vi "Emballage_BDD_lectureSQL_Liste PièceDansCmd.vi"(6 "order by":string="DATE_EMBALLAGE", 8 "Error in":errorcluster caption="Error in (no error)", 9 "Colonnes":string[](array[string])=["SN_PRODUIT\n", "DATE_EMBALLAGE\n", "ID_UTILISATEUR_GPAO\n", "NO_CDEVAL\n", "NO_DU_CARTON\n", "NO_RETOUR_CLIENT\n"], 10 "NO_CDEVAL":string="6340/07-02.01.01", 11 "Table (PRODUIT_EMBALLAGE)":string="PRODUIT_EMBALLAGE") -> (0 "Error out":errorcluster, 1 "Erreur de  comunication":bool, 2 "Liste n° pièces de la cmde":string[](array[string]), 3 "Donnees":string[][](array[string]), 4 "Carton":string[](array[string]))   [LabVIEW 2020]
uses:
  Modules/FS/60_FS_Controles/60_FS_SetGet.ctl
  <vilib>/addons/database/Connection.llb/DB Tools Open Connec (Path).vi
  <vilib>/addons/database/Connection.llb/Conn Execute.vi
  <vilib>/addons/database/Recordset.llb/Rec Fetch Recordset Data (R).vi
  <vilib>/addons/database/Recordset.llb/Rec Destroy - Connection.vi
  <vilib>/addons/database/NI_Database_API.lvlib
panel:
  out "temps Exe [s]":dbl
  in  "En cas de retour":string
  # "0"
  # "5"
  # "1"
  # "2"
  # "3"
  # "4"
  # "#LTI 20180802\nC'est quoi??\nvoir ancien et pas utiliser"
  # "0: SN_PRODUIT\n1: DATE_EMBALLAGE\n2: ID_UTILISATEUR_GPAO\n3: NO_CDEVAL\n4: NO_DU_CARTON\n5: NO_RETOUR_CLIENT"
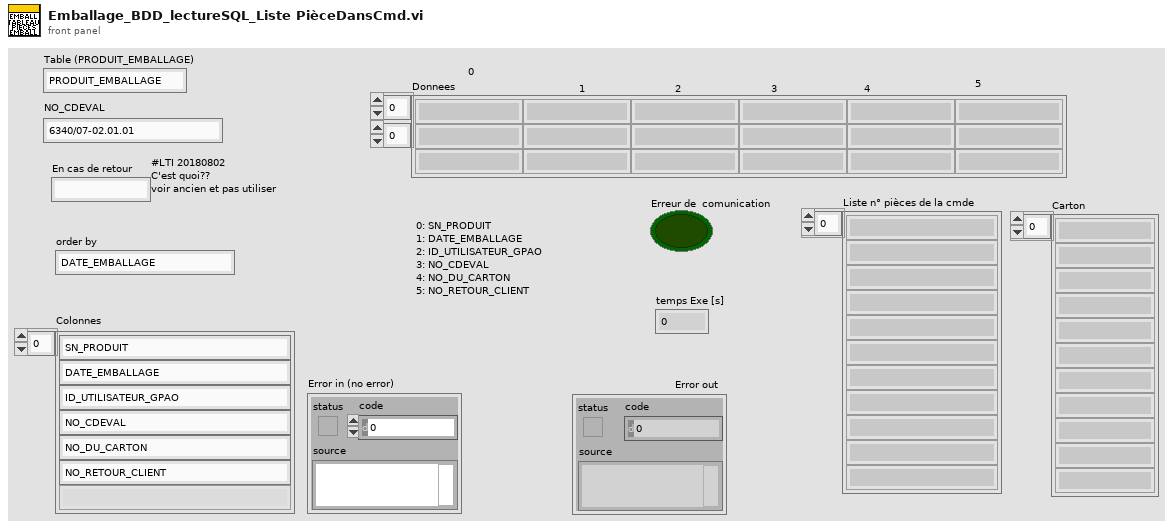
[diagram p1: front panel]
types:
  T1 = typedef "60_FS_SetGet.ctl" = enum16{"set", "get"}
  T2 = typedef "60_FS_CLT_Chemins.ctl" = cluster{"Racine_local":path, "Racine_reseau":path, "Racine_Support_Application":path, "Fichier_Journalisation":path, "Connexion_BDD_VSX":path, "Connexion_BDD_PLZ":path}
  T3 = typedef "NI_Database_API.lvlib/Conn ObjectReference.ctl" = refnum<k1>
  T4 = typedef "NI_Database_API.lvlib/Rec ObjectReference.ctl" = refnum<k1>
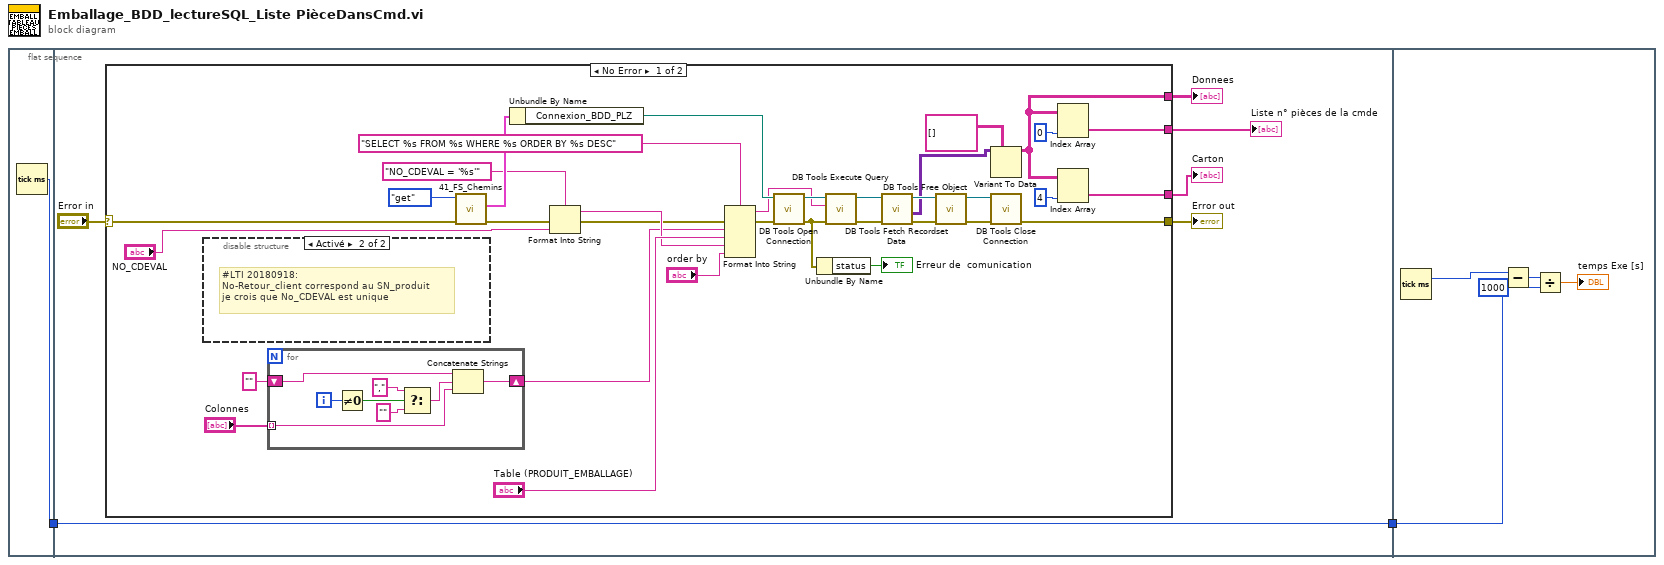
[diagram p0: block diagram]
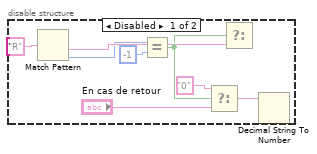
[diagram p2: hidden frame]
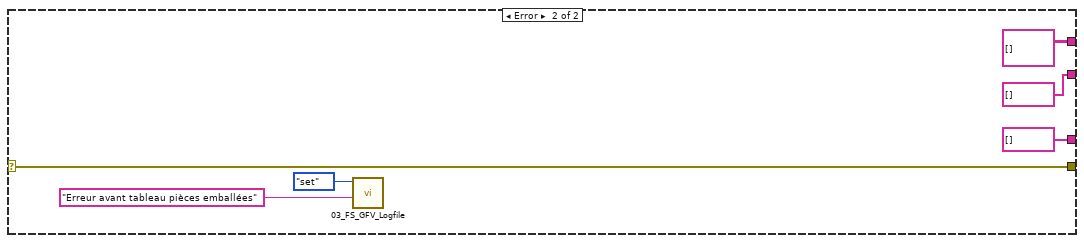
[diagram p3: hidden frame]
diagram:
  n1 = flat-sequence {
    tunnel: [w3] -> w2
    tunnel: w2 -> [w4]
    tunnel: [w4] -> w1
    tunnel: w1 -> [w66]
    frame #0 {
      n2 = Tick Count (ms)() -> (millisecond timer value=w3:u32)
    }
    frame #1 {
      n3 = case shown="No Error" "Error in" {
        selector: "Error in" -> [w29 w65]
        tunnel: [w28 w65] -> w8
        tunnel: [w12 string[][] [] ("Liste des champs à lire 2")] -> w7
        tunnel: [w14 string[] [] ("Liste des champs à lire 2")] -> w5
        tunnel: [w11 string[] [] ("Liste des champs à lire 2")] -> w6
        frame No Error {
          n4 = disable-structure shown="Activé" {
            frame Disabled {
              n5 = Match Pattern(regular expression="R" ("expression régulière")) -> (after substring=w51:string, offset past match=w49:i32)  [unwired: 2 in, 2 out]
              n6 = Equal?(x=w49, y=-1) -> (x = y?=w46:bool)
              n7 = Select(t="0", s=w46, f="En cas de retour") -> (s? t:f=w44:string)
              n8 = Select(s=w46, f=w51) -> ()  [unwired: 1 in, 1 out]
              n9 = Decimal String To Number(string=w44) -> ()  [unwired: 2 in, 2 out]
            }
            frame Enabled {
              # "#LTI 20180918:\nNo-Retour_client correspond au SN_produit\nje crois que No_CDEVAL est unique"
            }
          }
          n10 = for {
            tunnel: "Colonnes" -> [w58] mode=indexing
            shift-right: [w59] -> w19
            shift-left: "" -> [w57]
            i -> [w56]
            n11 = Not Equal To 0?(x=w56) -> (x != 0?=w55:bool)
            n12 = Select(t="," ("cas vrai"), s=w55, f="") -> (s? t:f=w54:string)
            n13 = Concatenate Strings(w57, w54, w58) -> (w59:string)
          }
          n14 = call "41_FS_Chemins.vi"("error in (no error)"=w29, "SetGet"=60_FS_SetGet."get") -> ("error out"=w31:errorcluster, "CLT_Chemins_out"=w39:T2)  [unwired: 8 in]
          n15 = Unbundle By Name(w39) -> ("Connexion_BDD_PLZ"=w37:path)
          n16 = Format Into String(format string="NO_CDEVAL = '%s'" ("chaîne de format"), error in=w31, "NO_CDEVAL") -> (resulting string=w33:string, error out=w30:errorcluster)  [unwired: 1 in]
          n17 = Format Into String(format string="SELECT %s FROM %s WHERE %s ORDER BY %s DESC" ("chaîne de format"), error in=w30, w19, "Table (PRODUIT_EMBALLAGE)", w33, "order by") -> (resulting string=w34:string, error out=w40:errorcluster)  [unwired: 1 in]
          n18 = call-poly <vilib>:"DB Tools Open Connection.vi"("error in (no error)"=w40, "connection information"=w37) -> ("error out"=w17:errorcluster, "connection reference"=w41:T3)  [unwired: 6 in]
          n19 = Unbundle By Name(w17) -> ("status"=→"Erreur de  comunication":bool)
          n20 = call-poly <vilib>:"DB Tools Execute Query.vi"("error in (no error)"=w17, "SQL query"=w34, "connection reference"=w41) -> ("error out"=w27:errorcluster, "recordset reference"=w25:T4)  [unwired: 5 in]
          n21 = call-poly <vilib>:"DB Tools Fetch Recordset Data.vi"("error in (no error)"=w27, "recordset reference"=w25) -> ("error out"=w26:errorcluster, "recordset data"=w23:variant[][], "recordset reference out"=w24:T4)  [unwired: 3 in]
          n22 = call-poly <vilib>:"DB Tools Free Object.vi"("error in (no error)"=w26, "recordset reference"=w24) -> ("error out"=w43:errorcluster, "connection reference"=w42:T3)  [unwired: 8 in]
          n23 = Variant To Data(type=string[][] [] ("Liste des champs à lire 2"), Variant=w23) -> (data=w12:string[][])  [unwired: 1 in, 1 out]
          n24 = call <vilib>:"DB Tools Close Connection.vi"("error in (no error)"=w43, "connection reference"=w42) -> ("error out"=w28:errorcluster)  [unwired: 5 in]
          n25 = Index Array(array=w12, index (col)=0 ("indice désactivé (col)")) -> (element=w14:string[])  [unwired: 1 in]
          n26 = Index Array(array=w12, index (col)=4 ("indice désactivé (col)")) -> (element=w11:string[])  [unwired: 1 in]
        }
        frame Error {
          n27 = call "03_FS_GFV_Logfile.vi"("Chaîne"="Erreur avant tableau pièces emballées", "States"=60_FS_SetGet."set") -> ()  [unwired: 8 in, 2 out]
        }
      }
      "Error out" <- w8
      "Donnees" <- w7
      "Liste n° pièces de la cmde" <- w5
      "Carton" <- w6
    }
    frame #2 {
      n28 = Tick Count (ms)() -> (millisecond timer value=w70:u32)
      n29 = Subtract(x=w70, y=w66) -> (x-y=w67:u32)
      n30 = Divide(x=w67, y=u32 1000) -> (x/y=→"temps Exe [s]":dbl)
    }
  }
